vi "ma_SML Spectrum (complex input).vi"(2 "FFT size":i32, 3 "window":u16(ring) items=["Rectangle"=0, "Hanning"=1, "Hamming"=2, "Blackman-Harris"=3, "Exact Blackman"=4, "Blackman"=5, "Flat Top"=6, "4 Term B-Harris "=7, "7 Term B-Harris"=8, "Low Sidelobe"=9, "Blackman Nuttall"=11, "Triangle"=30, "Bartlett-Hanning"=31, "Bohman"=32, "Parzen"=33, "Welch"=34, "Kaiser"=60, "Dolph-Chebyshev"=61, "Gaussian"=62], 4 "x [V]":cdb[](array[numeric]) format="%.2f") -> (0 "spectral info":T1 {"window" items=["Rectangle"=0, "Hanning"=1, "Hamming"=2, "Blackman-Harris"=3, "Exact Blackman"=4, "Blackman"=5, "Flat Top"=6, "4 Term B-Harris "=7, "7 Term B-Harris"=8, "Low Sidelobe"=9, "Blackman Nuttall"=11, "Triangle"=30, "Bartlett-Hanning"=31, "Bohman"=32, "Parzen"=33, "Welch"=34, "Kaiser"=60, "Dolph-Chebyshev"=61, "Gaussian"=62]}, 1 "FFT{x} [Vrms]":cdb[](array[numeric]) format="%.2f")   [LabVIEW 2020, in "NI_MAPro.lvlib"]
uses:
  NI_MAPro.lvlib
  ma_sml_Spectral Info.ctl
  NI_AALPro.lvlib
panel:
  # "complex signal's Windowed, normalized spectrum"
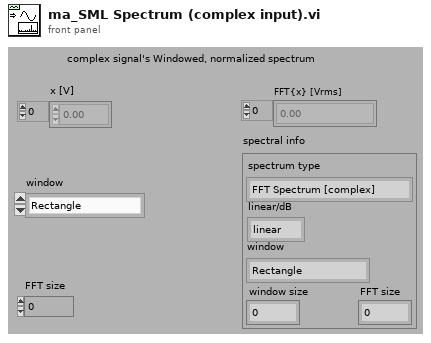
[diagram p1: front panel]
types:
  T1 = typedef "NI_MAPro.lvlib/ma_sml_Spectral Info.ctl" = cluster{"spectrum type":enum16{"FFT Spectrum [complex]", "Amplitude [Magnitude]", "Power [Magnitude^2]", "Cross Spectrum [complex]", "Frequency Response [Complex]"}, "linear/dB":enum16{"linear", "dB"}, "window":u16, "window size":i32, "FFT size":i32}
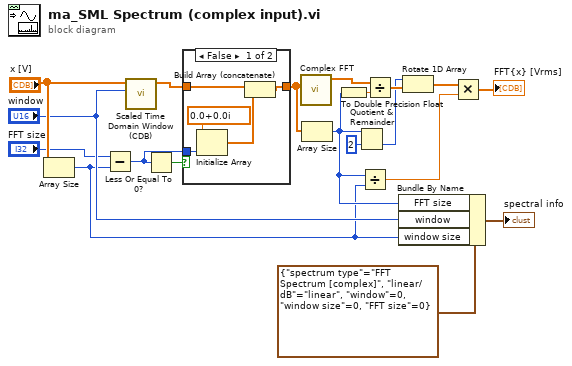
[diagram p0: block diagram]
diagram:
  n1 = Array Size(array="x [V]") -> (size(s)=w3:i32)
  n2 = Subtract(x="FFT size", y=w3) -> (x-y=w11:i32)
  n3 = call "Scaled Time Domain Window (CDB).vi"("window"="window", "X"="x [V]") -> ("Windowed X"=w14:cdb[])  [unwired: 7 in, 2 out]
  n4 = Less Or Equal To 0?(x=w11) -> (x <= 0?=w9:bool)
  n5 = case shown="False" w9 {
    tunnel: w14 -> [w21 w25]
    tunnel: [w22 w25] -> w13
    tunnel: w11 -> [w23 _]
    frame False {
      n6 = Initialize Array(cdb 0.0+0.0i ("Element Data"), w23) -> (w20:cdb[])
      n7 = Build Array (concatenate)(w21, w20) -> (w22:cdb[])
    }
    frame True {
    }
  }
  n8 = call "Complex FFT.vi"("X"=w13) -> ("FFT {X}"=w19:cdb[])  [unwired: 9 in, 1 out]
  n9 = Array Size(array=w13) -> (size(s)=w4:i32)
  n10 = To Double Precision Float(number=w4) -> (double precision float=w15:dbl)
  n11 = Quotient & Remainder(x=w4, y=2) -> (floor(x/y)=w16:i32)  [unwired: 1 out]
  n12 = Divide(x=w4, y=w3) -> (x/y=w2:dbl)
  n13 = Divide(x=w19, y=w15) -> (x/y=w18:cdb[])
  n14 = Bundle By Name(cluster=T1 {"spectrum type"=enum."FFT Spectrum [complex]", "linear/dB"=enum."linear", "window"=0, "window size"=0, "FFT size"=0} ("spectral info"), "FFT size"=w4, "window"="window", "window size"=w3) -> (→"spectral info":T1)
  n15 = Rotate 1D Array(1:w18, 2:w16) -> (0:w5:cdb[])
  n16 = Multiply(x=w5, y=w2) -> (x*y=→"FFT{x} [Vrms]":cdb[])
